vi "TDT-Set Trigger Val.vi"(0 "Data":T1={"TTankX"=refnum, "TDevAccX"=refnum, "LastTime"=0.0, "error"={"status"=FALSE, "code"=0, "source"=""}, "Block Name"="", "Circuit Tag"="", "Tank Name"="", "NumTicks"=0, "LastTick"=0.0, "Idle?"=FALSE, "Wait (ms)"=1000, "LastArtf"=0.0, "LastTosc"=0.0}, 7 "Val":dbl, 11 "error in (no error)":errorcluster) -> (15 "error out":errorcluster)   [LabVIEW 2015]
uses:
  TDT Interface Data.ctl
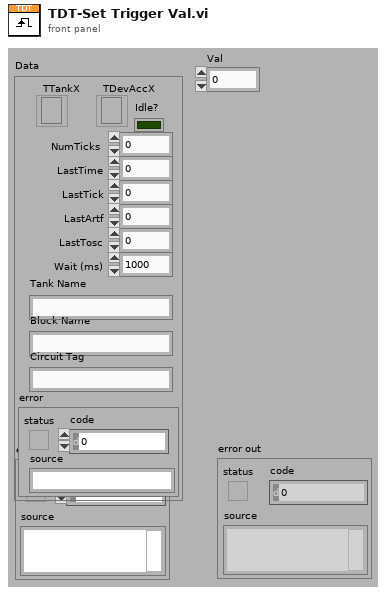
[diagram p1: front panel]
types:
  T1 = typedef "TDT Interface Data.ctl" = cluster{"TTankX":refnum<k7>, "TDevAccX":refnum<k7>, "LastTime":dbl, "error":errorcluster, "Block Name":string, "Circuit Tag":string, "Tank Name":string, "NumTicks":i32, "LastTick":dbl, "Idle?":bool, "Wait (ms)":u32, "LastArtf":dbl, "LastTosc":dbl}
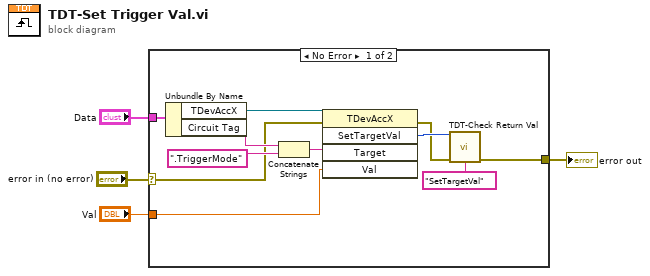
[diagram p0: block diagram]
diagram:
  n1 = case shown="No Error" "error in (no error)" {
    selector: "error in (no error)" -> [w8 w16]
    tunnel: "Val" -> [w7 _]
    tunnel: [w6 w16] -> w2
    tunnel: "Data" -> [w5 _]
    frame No Error {
      n2 = Unbundle By Name(w5) -> ("TDevAccX"=w15:refnum<k7>, "Circuit Tag"=w13:string)
      n3 = Concatenate Strings(w13, ".TriggerMode" ("string")) -> (w14:string)
      n4 = invoke class="TDevAccX" method="SetTargetVal"(reference=w15, error in=w8, "Target"=w14, "Val"=w7) -> (error out=w10:errorcluster, "SetTargetVal"=w11:i32)  [unwired: 1 in, 3 out]
      n5 = call "TDT-Check Return Val.vi"("Return Val"=w11, "error in (no error)"=w10, "source"="SetTargetVal" ("Message")) -> ("error out"=w6:errorcluster)  [unwired: 12 in]
    }
    frame Error {
    }
  }
  "error out" <- w2
